vi "test Value to String to Value (String).vi"(8 "error in":errorcluster, 11 "TestCase in":refnum<class "SharedUtilities.lvclass">) -> (0 "error out":errorcluster, 3 "TestCase out":refnum<class "SharedUtilities.lvclass">)   [LabVIEW 2020, in "SharedUtilities.lvclass"]
uses:
  SharedUtilities.lvclass
  0f61251e-6bce-40bc-9127-ed727464e5d8.vi
  a53efd5e-1b89-4488-9cb0-ebdcaa892606.vi
  4657b86e-0f3a-47b0-a768-c094f0f21e47.vi
  e7dd0ea7-1b51-4b32-9c58-6851ae4c1315.vi
  <vilib>/addons/_JKI Toolkits/VI Tester/TestCase.llb/TestCase.lvclass
  C:/Program Files (x86)/National Instruments/LabVIEW 2020/vi.lib/addons/_JKI Toolkits/VI Tester/TestCase.llb/TestCase.lvclass
  C:/Git/niveristand-ballard-milStd1553-custom-device/Source/Custom Device Support/Tests/Unit/Shared/SharedUtilities/SharedUtilities.lvclass
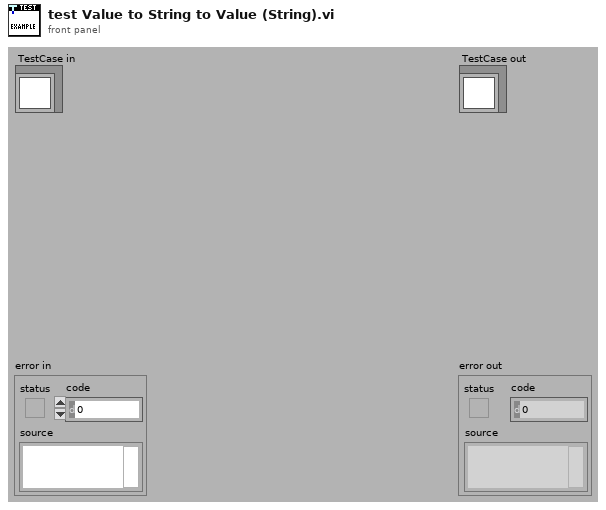
[diagram p1: front panel]
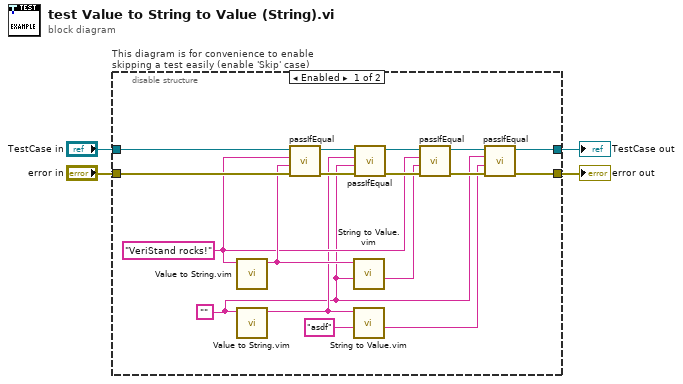
[diagram p0: block diagram]
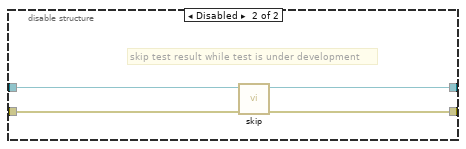
[diagram p2: hidden frame]
diagram:
  n1 = disable-structure "This diagram is for convenience to enable skipping a test easily (enable 'Skip' case)" shown="Enabled" {
    disable-tunnel: "TestCase in" -> [w11 w25]
    disable-tunnel: [w15 w23] -> w1
    disable-tunnel: [w14 w24] -> w3
    disable-tunnel: "error in" -> [w10 w22]
    frame Enabled {
      w7 = "VeriStand rocks!" ("string")
      w5 = ""
      n2 = call "Value to String.vim"("value"=w7) -> ("string"=w9:string)  [unwired: 10 in]
      n3 = call "Value to String.vim"("value"=w5) -> ("string"=w6:string)  [unwired: 10 in]
      n4 = call-dynamic "passIfEqual.vi"("error in (no error)"=w10, "y"=w9, "x"=w7, "TestCase in"=w11) -> ("error out"=w13:errorcluster, "TestCase out"=w12:refnum<class "SharedUtilities.lvclass">)  [unwired: 6 in]
      n5 = call "String to Value.vim"("default"=w5, "string"=w9) -> ("value"=w17:string)  [unwired: 9 in]
      n6 = call "String to Value.vim"("default"="asdf", "string"=w6) -> ("value"=w16:string)  [unwired: 9 in]
      n7 = call-dynamic "passIfEqual.vi"("error in (no error)"=w13, "y"=w5, "x"=w6, "TestCase in"=w12) -> ("error out"=w21:errorcluster, "TestCase out"=w20:refnum<class "SharedUtilities.lvclass">)  [unwired: 6 in]
      n8 = call-dynamic "passIfEqual.vi"("error in (no error)"=w21, "y"=w17, "x"=w7, "TestCase in"=w20) -> ("error out"=w19:errorcluster, "TestCase out"=w18:refnum<class "SharedUtilities.lvclass">)  [unwired: 6 in]
      n9 = call-dynamic "passIfEqual.vi"("error in (no error)"=w19, "y"=w16, "x"=w5, "TestCase in"=w18) -> ("error out"=w14:errorcluster, "TestCase out"=w15:refnum<class "SharedUtilities.lvclass">)  [unwired: 6 in]
    }
    frame Disabled {
      # "skip test result while test is under development"
      n10 = call <vilib>:"skip.vi"("error in (no error)"=w22, "TestCase in"=w25) -> ("error out"=w24:errorcluster, "TestCase out"=w23:refnum<class "SharedUtilities.lvclass">)  [unwired: 8 in]
    }
  }
  "error out" <- w3
  "TestCase out" <- w1
